vi "Drivetotarget.vi"() -> ()   [LabVIEW 2019]
uses:
  <vilib>/Rock Robotics/WPI/RobotDrive/WPI_RobotDriveArcadeDrive_Standard(NoSaturation).vi
  <vilib>/addons/control/pid/NI_PID_pid.lvlib
  <vilib>/addons/control/pid/pid.llb/PID (DBL).vi
panel:
  in  "PID gains":T1={"proportional gain (Kc)"=0.02, "integral time (Ti, min)"=0.0, "derivative time (Td, min)"=0.0} {"derivative time (Td, min)" format="%.3f"; "integral time (Ti, min)" format="%.3f"; "proportional gain (Kc)" format="%.3f"}
  out "output":dbl format="%.2f"
  in  "setpoint":dbl=5.0 format="%.2f"
  in  "PID gains 2":T1={"proportional gain (Kc)"=0.1, "integral time (Ti, min)"=0.01, "derivative time (Td, min)"=0.0} {"derivative time (Td, min)" format="%.3f"; "integral time (Ti, min)" format="%.3f"; "proportional gain (Kc)" format="%.3f"}
  out "ta":dbl
  out "tx":dbl
  out "tv":dbl
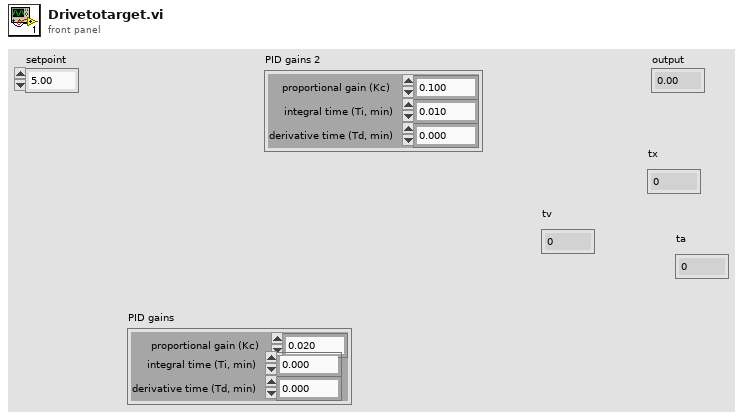
[diagram p1: front panel]
types:
  T1 = cluster{"proportional gain (Kc)":dbl, "integral time (Ti, min)":dbl, "derivative time (Td, min)":dbl}
  T2 = typedef "WPI_RobotDriveDevRef.ctl" = cluster{"DevStatus":errorcluster, "Motors[]":T3[], "Square Inputs":bool, "Max Output":dbl}
  T3 = typedef "WPI_MotorControlDeviceRef.ctl" = cluster{"DeviceStatus":errorcluster, "Type":T4, "PWM":cluster{"PWM Channel":T5, "DeadBand":T6}, "CAN":cluster{"Device Number":u8, "SetOutput VI Ref":variant, "GetOutput VI Ref":variant, "Enable VI Ref":variant, "Disable VI Ref":variant, "Data":variant}, "Invert":bool, "DIO PWM":cluster{"PWM \"Enable\" Channel":T5, "DIOChannel":T7, "PWM Rate":dbl}}
  T4 = typedef "WPI_MotorControlType.ctl" = enum16{"PWM", "CAN", "DIO PWM"}
  T5 = typedef "FPGA_DIOPWMChannel.ctl" = enum8{"PWM 0", "PWM 1", "PWM 2", "PWM 3", "PWM 4", "PWM 5", "PWM 6", "PWM 7", "PWM 8", "PWM 9", "PWM MXP 0", "PWM MXP 1", "PWM MXP 2", "PWM MXP 3", "PWM MXP 4", "PWM MXP 5", "PWM MXP 6", "PWM MXP 7", "PWM MXP 8", "PWM MXP 9", "Invalid"}
  T6 = typedef "WPI_PWMDeadband.ctl" = cluster{"Name":string, "maxPositivePwm":i32, "minPositivePwm":i32, "centerPwm":i32, "maxNegativePwm":i32, "minNegativePwm":i32, "angularRange":u16}
  T7 = typedef "FPGA_DIOChannel.ctl" = enum8{"DIO 0", "DIO 1", "DIO 2", "DIO 3", "DIO 4", "DIO 5", "DIO 6", "DIO 7", "DIO 8", "DIO 9", "DIO MXP 0", "DIO MXP 1", "DIO MXP 2", "DIO MXP 3", "DIO MXP 4", "DIO MXP 5", "DIO MXP 6", "DIO MXP 7", "DIO MXP 8", "DIO MXP 9", "DIO MXP 10", "DIO MXP 11", "DIO MXP 12", "DIO MXP 13", "DIO MXP 14", "DIO MXP 15", "SPI Port CS1", "SPI Port CS2", "SPI Port CS3", "SPI Port MISO", "SPI Port MOSI", "Invalid"}
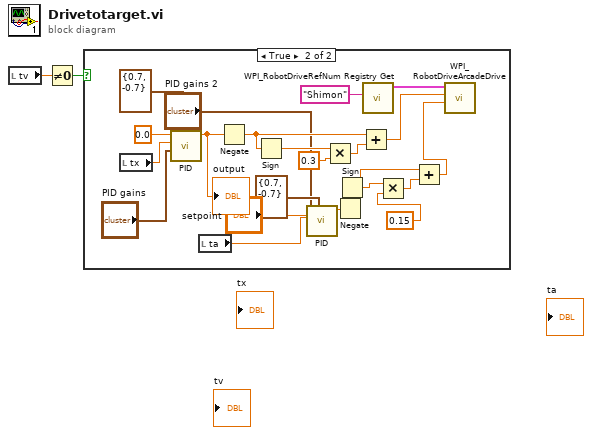
[diagram p0: block diagram]
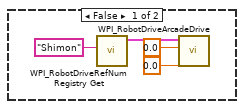
[diagram p2: hidden frame]
diagram:
  n1 = local read "tv"() -> (w2:dbl)
  n2 = Not Equal To 0?(x=w2) -> (x != 0?=w1:bool)
  n3 = case shown="True" w1 {
    frame False {
      n4 = call <vilib>:"WPI_RobotDriveRefNum Registry Get.vi"("refnum name"="Shimon") -> ("RobotDriveDevRef"=w6:T2)  [unwired: 9 in, 1 out]
      n5 = call-poly <vilib>:"WPI_RobotDriveArcadeDrive.vi"("Y axis value"=0.0, "X axis value"=0.0, "RobotDriveDevRef"=w6) -> ()  [unwired: 6 in, 3 out]
    }
    frame True {
      n6 = local read "tx"() -> (w25:dbl)
      n7 = call-poly <vilib>:"PID.vi"("output range"=cluster{"output high":dbl, "output low":dbl} {"output high"=0.7, "output low"=-0.7}, "PID gains"="PID gains", "process variable"=w25, "setpoint"=0.0) -> ("output"=w26:dbl)  [unwired: 6 in, 1 out]
      "output" <- w26
      n8 = local read "ta"() -> (w14:dbl)
      n9 = Negate(x=w26) -> (-x=w18:dbl)
      n10 = Sign(1:w18) -> (0:w21:dbl)
      n11 = call-poly <vilib>:"PID.vi"("output range"=cluster{"output high":dbl, "output low":dbl} {"output high"=0.7, "output low"=-0.7}, "PID gains"="PID gains 2", "process variable"=w14, "setpoint"="setpoint") -> ("output"=w10:dbl)  [unwired: 6 in, 1 out]
      n12 = Multiply(x=w21, y=0.3) -> (x*y=w19:dbl)
      n13 = Negate(x=w10) -> (-x=w7:dbl)
      n14 = Sign(1:w7) -> (0:w8:dbl)
      n15 = Add(x=w18, y=w19) -> (x+y=w17:dbl)
      n16 = call <vilib>:"WPI_RobotDriveRefNum Registry Get.vi"("refnum name"="Shimon") -> ("RobotDriveDevRef"=w28:T2)  [unwired: 9 in, 1 out]
      n17 = Multiply(x=w8, y=0.15 ("Y axis value")) -> (x*y=w12:dbl)
      n18 = Add(x=w7, y=w12) -> (x+y=w9:dbl)
      n19 = call-poly <vilib>:"WPI_RobotDriveArcadeDrive.vi"("Y axis value"=w9, "X axis value"=w17, "RobotDriveDevRef"=w28) -> ()  [unwired: 6 in, 3 out]
    }
  }
